vi "CRYBoxcar Median Keep-Len.vi"(10 "Rank":i32, 11 "Measured curve":dbl[](array[numeric]) format="%.2f") -> (3 "Smoothed curve":dbl[](array[numeric]) format="%.2f")   [LabVIEW 2013]
doc: "General-purpose boxcar averaging for float arrays. Rank input is the number of points to average in from each side of the data point. For instance, a Rank of 2 makes a sliding boxcar of size 5. The resulting \"Smoothed curve\" array is 2 X Rank shorter than the input \"Measured curve.\""
uses:
  <vilib>/Analysis/NI_AALBase.lvlib
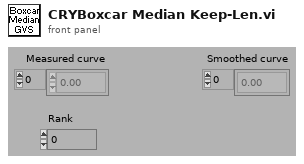
[diagram p1: front panel]
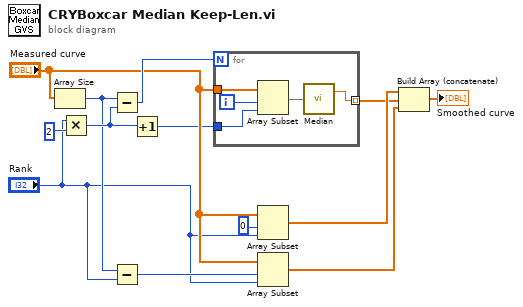
[diagram p0: block diagram]
diagram:
  n1 = Array Size(array="Measured curve") -> (size(s)=w8:i32)
  n2 = Multiply(x="Rank", y=2) -> (x*y=w11:i32)
  n3 = Subtract(x=w8, y=w11) -> (x-y=w12:i32)
  n4 = Subtract(x=w8, y="Rank") -> (x-y=w7:i32)
  n5 = Increment(x=w11) -> (x+1=w2:i32)
  n6 = for {
    N: w12 -> [_]
    tunnel: w2 -> [w17]
    tunnel: "Measured curve" -> [w16]
    tunnel: [w14] -> w1 mode=indexing
    i -> [w18]
    n7 = Array Subset(array=w16, index=w18, length=w17) -> (w15:dbl[])
    n8 = call <vilib>:"Median.vi"("X"=w15) -> ("median"=w14:dbl)  [unwired: 1 out]
  }
  n9 = Array Subset(array="Measured curve", index=0, length="Rank") -> (w4:dbl[])
  n10 = Array Subset(array="Measured curve", index=w7, length="Rank") -> (w5:dbl[])
  n11 = Build Array (concatenate)(w4, w1, w5) -> (→"Smoothed curve":dbl[])
